vi "Create RT Sequence.vi"(8 "error in (no error)":errorcluster, 11 "RT Sequence Path":path) -> (0 "error out":errorcluster, 3 "RT Sequence Ref":refnum<k24>)   [LabVIEW 2016, in "RT Sequence Creator API.lvlib"]
uses:
  RT Sequence Creator API.lvlib
  NationalInstruments.VeriStand.RealTimeSequenceDefinitionApi
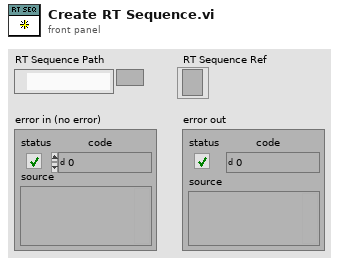
[diagram p1: front panel]
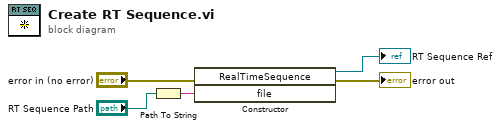
[diagram p0: block diagram]
diagram:
  n1 = Path To String(path="RT Sequence Path") -> (string=w3:string)
  n2 = constructor class="RealTimeSequence"(error in="error in (no error)", "file"=w3) -> (reference out=→"RT Sequence Ref":refnum<k24>, error out=→"error out":errorcluster)  [unwired: 2 in, 2 out]
